vi "CRC_compare.vi"(8 "error in":errorcluster, 11 "array_in":u8[](array[numeric])) -> (0 "error out":errorcluster, 1 "Plot_T":bool, 2 "array_out":u8[](array[numeric]), 3 "CRC":bool)   [LabVIEW 2017]
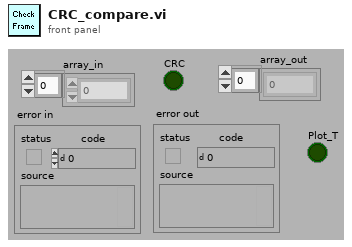
[diagram p1: front panel]
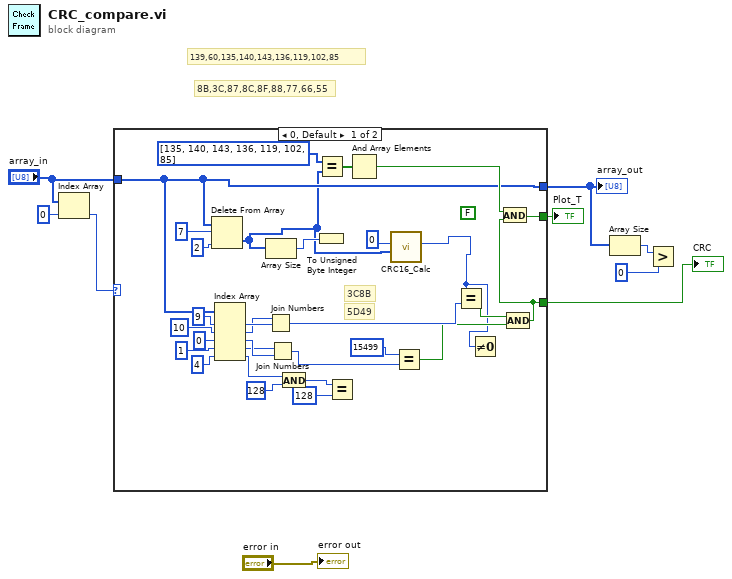
[diagram p0: block diagram]
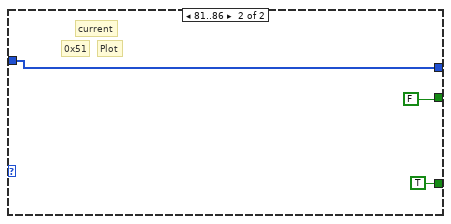
[diagram p2: hidden frame]
diagram:
  # "8B,3C,87,8C,8F,88,77,66,55"
  # "139,60,135,140,143,136,119,102,85"
  n1 = Index Array(array="array_in", index=0) -> (element=w6:u8)
  n2 = case shown="0, Default" w6 {
    tunnel: [w14 TRUE] -> w1
    tunnel: [w13 w41] -> w4
    tunnel: "array_in" -> [w13 w41]
    tunnel: [w16 FALSE] -> w5
    frame 0, Default {
      (unwired) FALSE
      # "5D49"
      # "3C8B"
      n3 = Delete From Array(array=w13, length=7, index=2) -> (deleted portion=w12:u8[])  [unwired: 1 out]
      n4 = Index Array(array=w13, index #1=9 ("index"), index #2=10 ("index"), index #3=0 ("index"), index #4=1 ("index"), index #5=4 ("index")) -> (element #1=w34:u8, element #2=w33:u8, element #3=w29:u8, element #4=w28:u8, element #5=w24:u8)
      n5 = Array Size(array=w12) -> (size(s)=w39:i32)
      n6 = Join Numbers(hi=w33, lo=w34) -> ((hi.lo)=w30:u16)
      n7 = Join Numbers(hi=w28, lo=w29) -> ((hi.lo)=w27:u16)
      n8 = And(x=w24, y=u8 128) -> (x .and. y?=w21:u8)
      n9 = To Unsigned Byte Integer(number=w39) -> ()  [unwired: 1 out]
      n10 = Equal?(x=u8[] [135, 140, 143, 136, 119, 102, 85], y=w12) -> (x = y?=w19:bool[])
      n11 = Equal?(x=w21, y=u8 128) -> ()  [unwired: 1 out]
      n12 = And Array Elements(Boolean array=w19) -> (logical AND=w15:bool)
      n13 = call "CRC16_Calc.vi"("buffer"=w12, "crc"=u16 0 ("CRC")) -> ("crc 2"=w11:u16)  [unwired: 9 in]
      n14 = Equal?(x=u16 15499, y=w27) -> (x = y?=w17:bool)
      n15 = Equal?(x=w11, y=w30) -> (x = y?=w18:bool)
      n16 = Not Equal To 0?(x=w11) -> ()  [unwired: 1 out]
      n17 = Compound Arithmetic op=AND(w18, w17) -> (w14:bool)
      n18 = And(x=w15, y=w14) -> (x .and. y?=w16:bool)
    }
    frame 81..86 {
      # "current"
      # "Plot"
      # "0x51"
    }
  }
  "CRC" <- w1
  "array_out" <- w4
  "Plot_T" <- w5
  n19 = Array Size(array=w4) -> (size(s)=w3:i32)
  n20 = Greater?(x=w3, y=0) -> ()  [unwired: 1 out]
  "error out" <- "error in"
